vi "Referect_EnableCh_for_form.vi"(8 "错误输入（无错误）":errorcluster, 10 "MPM":refnum<k24>[](array[refnum]), 11 "数组输入":bool[](array[boolean])) -> (0 "error IO":errorcluster, 3 "数组输出":bool[](array[boolean]))   [LabVIEW 2017]
uses:
  D:/test/ILSTS/LV_IL/LV_IL_Sample_x86/DLL/InstrumentDLL.dll
  DLL/InstrumentDLL.dll
  Share/PowerMonitorType.vi
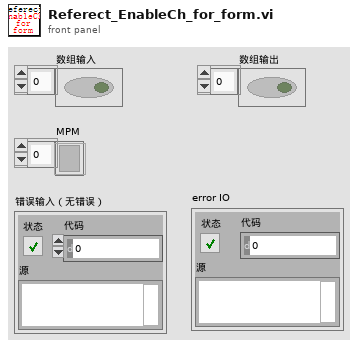
[diagram p1: front panel]
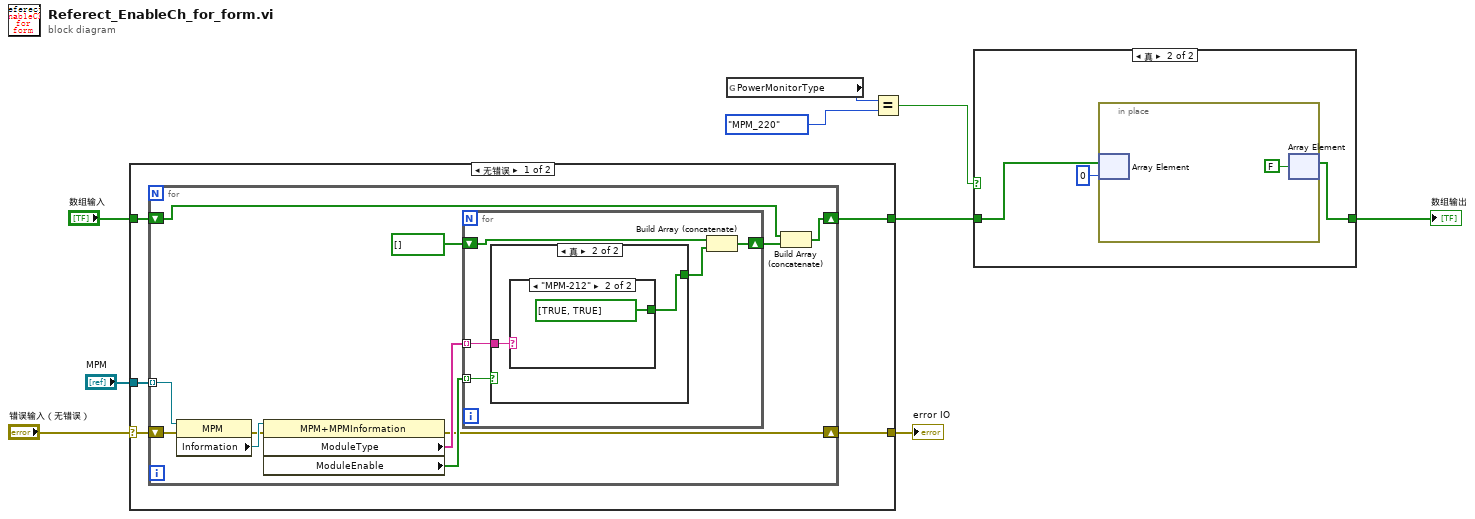
[diagram p0: block diagram]
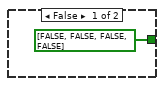
[diagram p3: hidden frame]
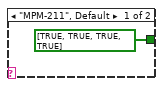
[diagram p4: hidden frame]
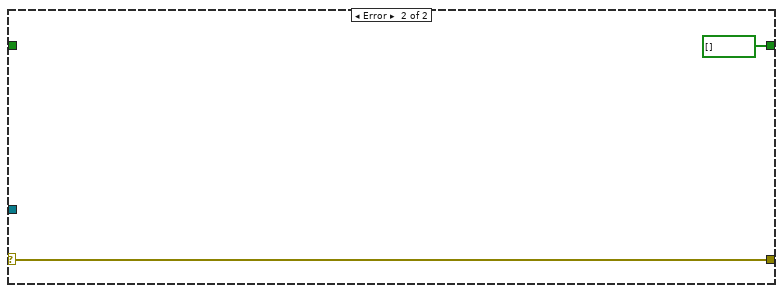
[diagram p5: hidden frame]
diagram:
  n1 = case shown="无错误" "错误输入（无错误）" {
    selector: "错误输入（无错误）" -> [w11 w36]
    tunnel: [w14 bool[] [] ("数组输入")] -> w2
    tunnel: "数组输入" -> [w13 _]
    tunnel: "MPM" -> [w12 _]
    tunnel: [w10 w36] -> w6
    frame No Error {
      n2 = for {
        tunnel: w12 -> [w24] mode=indexing
        shift-right: [w18] -> w14
        shift-left: w13 -> [w22]
        shift-right: [w15] -> w10
        shift-left: w11 -> [w17]
        n3 = property on="属性节点" class="MPM"(reference=w24, error in=w17) -> (error out=w16:errorcluster, "Information"=w25:refnum<k24>)  [unwired: 1 out]
        n4 = property class="MPM+MPMInformation"(reference=w25, error in=w16) -> (error out=w15:errorcluster, "ModuleType"=w23:string[], "ModuleEnable"=w19:bool[])  [unwired: 1 out]
        n5 = for {
          tunnel: w23 -> [w30] mode=indexing
          shift-right: [w27] -> w20
          shift-left: bool[] [] ("添加的数组") -> [w28]
          tunnel: w19 -> [w26] mode=indexing
          n6 = case shown="真" w26 {
            tunnel: w30 -> [_ w33]
            tunnel: [bool[] [FALSE, FALSE, FALSE, FALSE] w32] -> w29
            frame False {
            }
            frame True {
              n7 = case shown="\"MPM-212\"" w33 {
                tunnel: [bool[] [TRUE, TRUE, TRUE, TRUE] bool[] [TRUE, TRUE]] -> w32
                frame "MPM-211", Default {
                }
                frame "MPM-212" {
                }
              }
            }
          }
          n8 = Build Array (concatenate)(w28, w29) -> (w27:bool[])
        }
        n9 = Build Array (concatenate)(w22, w20) -> (w18:bool[])
      }
    }
    frame Error {
    }
  }
  "error IO" <- w6
  n10 = global read "PowerMonitorType.vi" "PowerMonitorType"() -> (w5:enum16{"DAQ", "MPM_220", "TSL_LOGG"})
  n11 = Equal?(x=w5, y=enum16{"DAQ", "MPM_220", "TSL_LOGG"}."MPM_220") -> (x = y?=w3:bool)
  n12 = case shown="真" w3 {
    tunnel: w2 -> [w38 w41]
    tunnel: [w38 w39] -> w1
    frame False {
    }
    frame True {
      n13 = in-place {
        n14 = in-place-array #1(w41, 0) -> ()  [unwired: 1 out]
        n15 = in-place-array #1(FALSE ("element")) -> (w39:bool[])  [unwired: 1 out]
      }
    }
  }
  "数组输出" <- w1
